vi "Perform Ch To Ch Isolation Measurement.vi"(8 "error in":errorcluster, 10 "Measurement Results in":T1, 11 "ananlog waveforms":waveform(dbl)[](array[waveform])) -> (0 "error out":errorcluster, 2 "Measurement Results out":T1)   [LabVIEW 2021, in "Channel To Channel Isolation_ADC.lvlib"]
uses:
  Channel To Channel Isolation_ADC.lvlib
  Measurement Results.ctl
  <vilib>/addons/_NISVFA/_Shared subVIs/Controls/svc_Window.ctl
  <vilib>/addons/_NISVFA/_Spectrum Processing/SVFA Unit Conversion (Complex) (N Ch).vi
  <vilib>/addons/_NISVFA/_Spectrum Processing/SVFA Unit Conversion (Complex) (1 Ch).vi
  <vilib>/addons/_NISVFA/_Shared subVIs/Common/svc_Log View for Spectrum (1Ch).vi
  <vilib>/addons/_NISVFA/_Spectrum Processing/SVFA Unit Conversion (1 Ch).vi
  <vilib>/addons/_NISVFA/_Shared subVIs/Common/svc_Complex Datatype Defaults.vi
  <vilib>/addons/_NISVFA/_Shared subVIs/Common/svc_Unwrap Phase.vi
  <vilib>/addons/_NISVFA/_Shared subVIs/Common/svc_Convert Spectrum Array to dB.vi
  <vilib>/addons/_NISVFA/_Shared subVIs/Common/svc_Spectrum Units.vi
  <vilib>/addons/_NISVFA/_Spectrum Processing/subVIs/svfa_Conversion Utility (spectrum info).vi
  <vilib>/addons/_NISVFA/_Shared subVIs/Common/svc_Format Value (DBL).vi
  <vilib>/addons/_NISVFA/_Shared subVIs/Common/svc_Get Weighting Enum and Labels.vi
  <vilib>/addons/_NISVFA/_Shared subVIs/Common/svc_Engineering Units to Unit Label.vi
  <vilib>/addons/_NISVFA/_Shared subVIs/Common/svc_Surround NonAlpha String with Parentheses.vi
  <vilib>/dlg_ctls.llb/Space Constant.vi
  <vilib>/addons/_NISVFA/_Spectrum Processing/subVIs/svfa_Peak to RMS to Peak2Peak.vi
  <vilib>/addons/_NISVFA/_Spectrum Processing/subVIs/svfa_Mag to Mag2.vi
  <vilib>/addons/_NISVFA/_Spectrum Processing/subVIs/svfa_Linear to dB.vi
  <vilib>/addons/_NISVFA/_Spectrum Processing/subVIs/svfa_dBrefA to dBrefB.vi
  <vilib>/addons/_NISVFA/_Spectrum Processing/subVIs/svfa_Spectrum to Spectral Density.vi
  <vilib>/addons/_NISVFA/_Shared subVIs/Common/svc_Unit Label Lexical Class.vi
  <vilib>/addons/_NISVFA/_Shared subVIs/Common/svc_Window Parameters.vi
  <vilib>/Analysis/4window.llb/window parameters.vi
  <vilib>/Analysis/4window.llb/Window Properties.vi
  <vilib>/Analysis/4window.llb/Window Properties by Name.vi
  <vilib>/addons/_NISVFA/_Shared subVIs/Common/svc_Caller VI Returned in Error Source.vi
  <vilib>/addons/Sound and Vibration/svt_Single Tone Measurements/SoundVib_SingleTone.lvlib
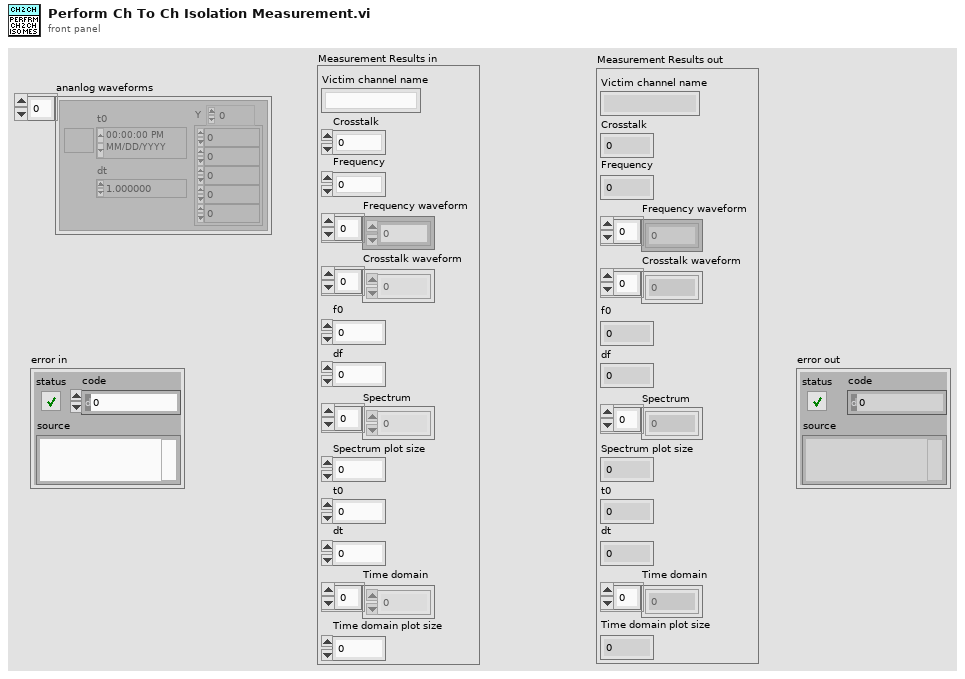
[diagram p1: front panel]
types:
  T1 = typedef "Channel To Channel Isolation_ADC.lvlib/Measurement Results.ctl" = cluster{"Victim channel name":string, "Crosstalk":dbl, "Frequency":dbl, "Frequency waveform":dbl[], "Crosstalk waveform":dbl[], "f0":dbl, "df":dbl, "Spectrum":dbl[], "Spectrum plot size":i32, "t0":dbl, "dt":dbl, "Time domain":dbl[], "Time domain plot size":i32}
  T2 = typedef "svc_Window.ctl" = u32
  T3 = cluster{"linear/dB":enum16{"no change", "linear", "dB"}, "dB reference (0: no change)":dbl, "power/magnitude":enum16{"no change", "power", "magnitude"}, "view":enum16{"no change", "rms", "peak", "peak-peak"}}
  T4 = typedef "svc_Spectrum Info.ctl" = cluster{"channel name":string, "description":string, "x-axis units":T5, "spectral info":cluster{"spectrum type":T6, "linear/dB":enum16{"linear", "dB"}, "window":u16, "window size":i32, "FFT size":i32}, "engineering units":T7, "custom label":string, "dB reference [EU]":dbl, "peak units":enum16{"rms", "peak", "peak-peak"}, "weighting filter":T8, "spectral density?":bool, "unit label":string, "spectrum skewed?":bool, "complimentary spectrum units":T9}
  T5 = typedef "svc_X-Axis Units.ctl" = u16
  T6 = typedef "svc_Spectrum Type.ctl" = enum16{"FFT Spectrum [complex]", "Amplitude [Magnitude]", "Power [Magnitude^2]", "Cross Spectrum [complex]", "Frequency Response [Complex]"}
  T7 = typedef "svc_Engineering Units Text Ring.ctl" = u16
  T8 = typedef "svc_Weighting Filter Text Ring.ctl" = u16
  T9 = typedef "svc_Complimentary Spectrum Units.ctl" = enum16{"none", "radians", "degrees", "cycles", "imaginary"}
  T10 = cluster{"complex spectrum response":cluster{"f0":dbl, "df":dbl, "complex spectrum":cdb[]}, "spectrum info":T4}
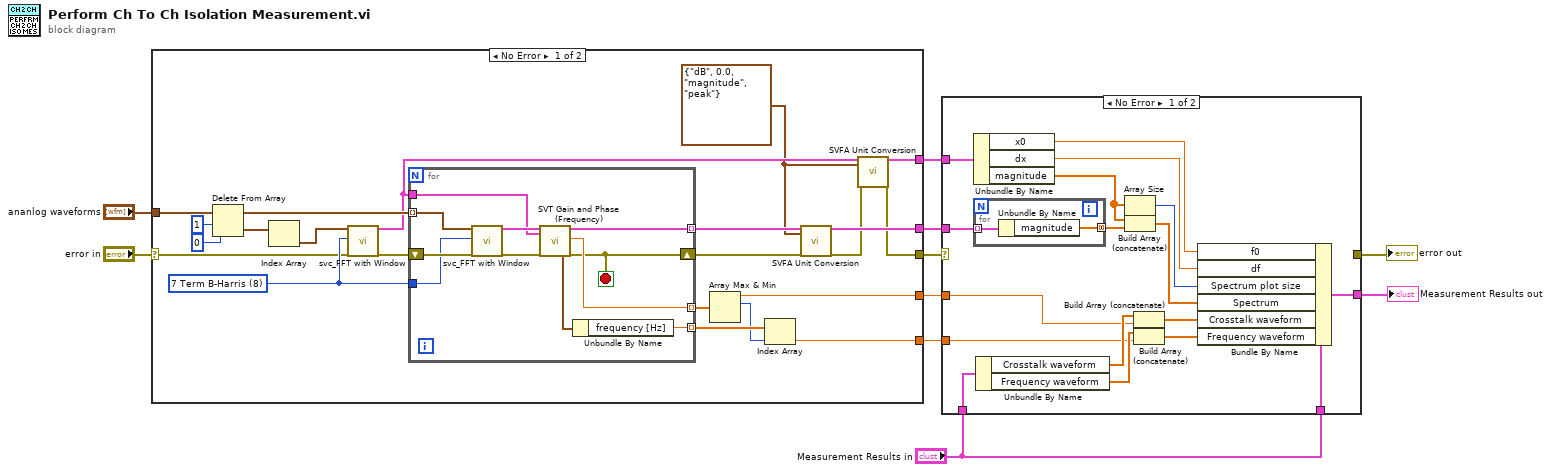
[diagram p0: block diagram]
diagram:
  n1 = case shown="No Error" "error in" {
    selector: "error in" -> [w21 w43]
    tunnel: [w15 w43] -> w8
    tunnel: "ananlog waveforms" -> [w30 _]
    tunnel: [w20 _] -> w7
    tunnel: [w19 _] -> w6
    tunnel: [w18 _] -> w2
    tunnel: [w14 _] -> w3
    frame No Error {
      w29 = T2 8 items=["None ", "Hanning", "Hamming", "Blackman-Harris", "Exact Blackman", "Blackman", "Flat Top", "4 Term B-Harris ", "7 Term B-Harris", "Low Sidelobe"] ("window")
      w13 = T3 {"linear/dB"=enum."dB", "dB reference (0: no change)"=0.0, "power/magnitude"=enum."magnitude", "view"=enum."peak"} ("desired scaling")
      n2 = Delete From Array(array=w30, length=1, index=0) -> (deleted portion=w12:waveform(dbl)[], array with subset deleted=w25:waveform(dbl)[])
      n3 = Index Array(array=w12) -> (element=w11:waveform(dbl))  [unwired: 1 in]
      n4 = call <vilib>:"svc_FFT with Window.vi"("time signal in [EU]"=w11, "window"=w29, "error in"=w21) -> ("complex spectrum"=w17:T10, "error out"=w28:errorcluster)  [unwired: 15 in]
      n5 = for {
        tunnel: [w39] -> w32 mode=indexing
        shift-right: [w34] -> w31
        shift-left: w28 -> [w42]
        tunnel: w29 -> [w41]
        tunnel: w25 -> [w40] mode=indexing
        tunnel: w17 -> [w33]
        tunnel: [w37] -> w24 mode=indexing
        tunnel: [w35] -> w23 mode=indexing
        stop <- w34 stop-if-true
        n6 = call <vilib>:"svc_FFT with Window.vi"("time signal in [EU]"=w40, "window"=w41, "error in"=w42) -> ("complex spectrum"=w39:T10, "error out"=w38:errorcluster)  [unwired: 15 in]
        n7 = call <vilib>:"SVT Gain and Phase (Frequency).vi"("complex spectrum\nstimulus X"=w39, "complex spectrum\nresponse Y"=w33, "error in (no error)"=w38) -> ("detected tone stimulus"=w36:cluster{"frequency [Hz]":dbl, "amplitude":dbl}, "gain"=w37:dbl, "error out"=w34:errorcluster)  [unwired: 9 in, 5 out]
        n8 = Unbundle By Name(w36) -> ("frequency [Hz]"=w35:dbl)
      }
      n9 = Array Max & Min(array=w24) -> (max value=w20:dbl, max index (indices)=w22:i32)  [unwired: 2 out]
      n10 = Index Array(array=w23, index=w22) -> (element=w19:dbl)
      n11 = call-poly <vilib>:"SVFA Unit Conversion.vi"("complex spectra"=w32, "desired scaling"=w13, "error in (no error)"=w31) -> ("converted spectra"=w18:cluster{"x0":dbl, "dx":dbl, "magnitude":dbl[]}[], "error out"=w16:errorcluster)  [unwired: 11 in, 4 out]
      n12 = call-poly <vilib>:"SVFA Unit Conversion.vi"("complex spectrum"=w17, "desired scaling"=w13, "error in (no error)"=w16) -> ("converted spectrum"=w14:cluster{"x0":dbl, "dx":dbl, "magnitude":dbl[]}, "error out"=w15:errorcluster)  [unwired: 11 in, 4 out]
    }
    frame Error {
    }
  }
  n13 = case shown="No Error" w8 {
    selector: w8 -> [_ w63]
    tunnel: "Measurement Results in" -> [w60 _]
    tunnel: w7 -> [w57 _]
    tunnel: w6 -> [w55 _]
    tunnel: "Measurement Results in" -> [w59 _]
    tunnel: [w52 _] -> w4
    tunnel: w3 -> [w51 _]
    tunnel: w2 -> [w50 _]
    tunnel: [_ w63] -> w1
    frame No Error {
      n14 = Unbundle By Name(w51) -> ("x0"=w48:dbl, "dx"=w47:dbl, "magnitude"=w46:dbl[])
      n15 = for {
        tunnel: w50 -> [w62] mode=indexing
        tunnel: [w61] -> w49 mode=concatenating
        n16 = Unbundle By Name(w62) -> ("magnitude"=w61:dbl[])
      }
      n17 = Unbundle By Name(w59) -> ("Crosstalk waveform"=w58:dbl[], "Frequency waveform"=w56:dbl[])
      n18 = Array Size(array=w46) -> (size(s)=w45:i32)
      n19 = Build Array (concatenate)(w46, w49) -> (w44:dbl[])
      n20 = Build Array (concatenate)(w58, w57) -> (w53:dbl[])
      n21 = Build Array (concatenate)(w56, w55) -> (w54:dbl[])
      n22 = Bundle By Name(cluster=w60, "f0"=w48, "df"=w47, "Spectrum plot size"=w45, "Spectrum"=w44, "Crosstalk waveform"=w53, "Frequency waveform"=w54) -> (w52:T1)
    }
    frame Error {
    }
  }
  "error out" <- w1
  "Measurement Results out" <- w4
